vi "_046.vi"() -> ()   [LabVIEW 2024]
panel:
  out "length":i32
  in  "Numeric":i64
  # "Digit Count from Integer :"
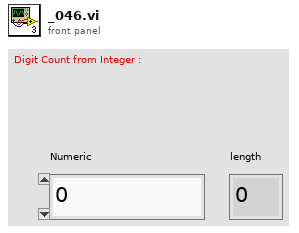
[diagram p1: front panel]
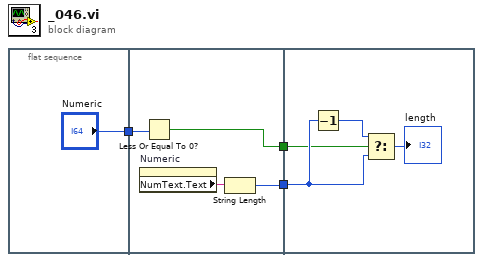
[diagram p0: block diagram]
diagram:
  n1 = flat-sequence {
    tunnel: ["Numeric"] -> w3
    tunnel: w3 -> [w8]
    tunnel: [w6] -> w2
    tunnel: [w5] -> w1
    tunnel: w2 -> [w11]
    tunnel: w1 -> [w9]
    frame #0 {
    }
    frame #1 {
      n2 = property on="Numeric" class="DigNum (strict)"() -> ("NumText.Text"=w7:string)  [unwired: 2 in, 2 out]
      n3 = Less Or Equal To 0?(x=w8) -> (x <= 0?=w5:bool)
      n4 = String Length(string=w7) -> (length=w6:i32)
    }
    frame #2 {
      n5 = Decrement(x=w11) -> (x-1=w10:i32)
      n6 = Select(t=w10, s=w9, f=w11) -> (s? t:f=→"length":i32)
    }
  }
